vi "Read VI Interpreter.vi"(9 "RasPi Compiler in":refnum<class "RasPi Compiler.lvclass">) -> (3 "RasPi Compiler out":refnum<class "RasPi Compiler.lvclass">, 4 "VI Interpreter":refnum<class "VI Interpreter.lvclass">)   [LabVIEW 2014, in "RasPi Compiler.lvclass"]
uses:
  RasPi Compiler.lvclass
  VI Interpreter/Classes/VI Interpreter/VI Interpreter.lvclass
  RasPi Compiler.lvclass/RasPi Compiler.ctl
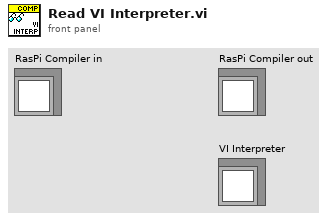
[diagram p1: front panel]
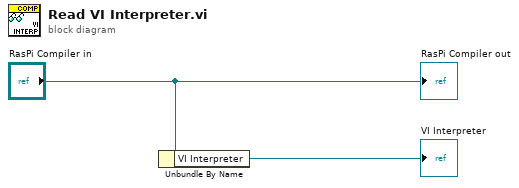
[diagram p0: block diagram]
diagram:
  n1 = Unbundle By Name("RasPi Compiler in") -> ("VI Interpreter"=→"VI Interpreter":refnum<class "VI Interpreter.lvclass">)
  "RasPi Compiler out" <- "RasPi Compiler in"
